vi "Identify.vi"(8 "error in (no error)":errorcluster, 11 "BML Pattern Creater in":refnum<class "BML Pattern Creater.lvclass">) -> (0 "error out":errorcluster, 2 "Plugin is Valid":bool, 3 "BML Pattern Creater out":refnum<class "BML Pattern Creater.lvclass">)   [LabVIEW 2018, in "BML Pattern Creater.lvlib" / "BML Pattern Creater.lvclass"]
uses:
  BML Pattern Creater.lvclass
  Interfaces/Protocol Interface.lvlibp/Interfaces/Protocol Interface/Protocol Interface.lvclass
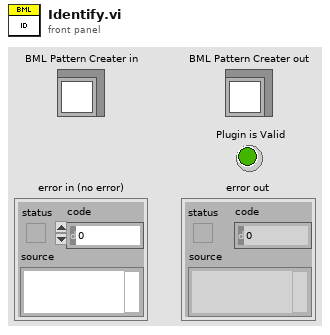
[diagram p1: front panel]
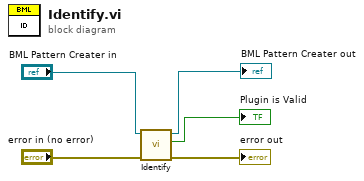
[diagram p0: block diagram]
diagram:
  n1 = call-parent "Identify.vi"("error in (no error)"="error in (no error)", "Protocol Interface in"="BML Pattern Creater in") -> ("error out"=→"error out":errorcluster, "Plugin is Valid"=→"Plugin is Valid":bool, "Protocol Interface out"=→"BML Pattern Creater out":refnum<class "BML Pattern Creater.lvclass">)  [unwired: 7 in]
